vi "CANFD Frame to std frm.vi"(1 "Channel":i32, 3 "CANFD Frame":T2(array[cluster])) -> (0 "CAN Std Frm":T1[](array[typedef]) {"Direction" items=["Tx", "Rx"]; "CANType" items=["CAN", "CANFD", "CANFD加速"]})   [LabVIEW 2018, in "CAN FD.lvlib"]
uses:
  CAN FD.lvlib
  Typedef/CAN Data.ctl
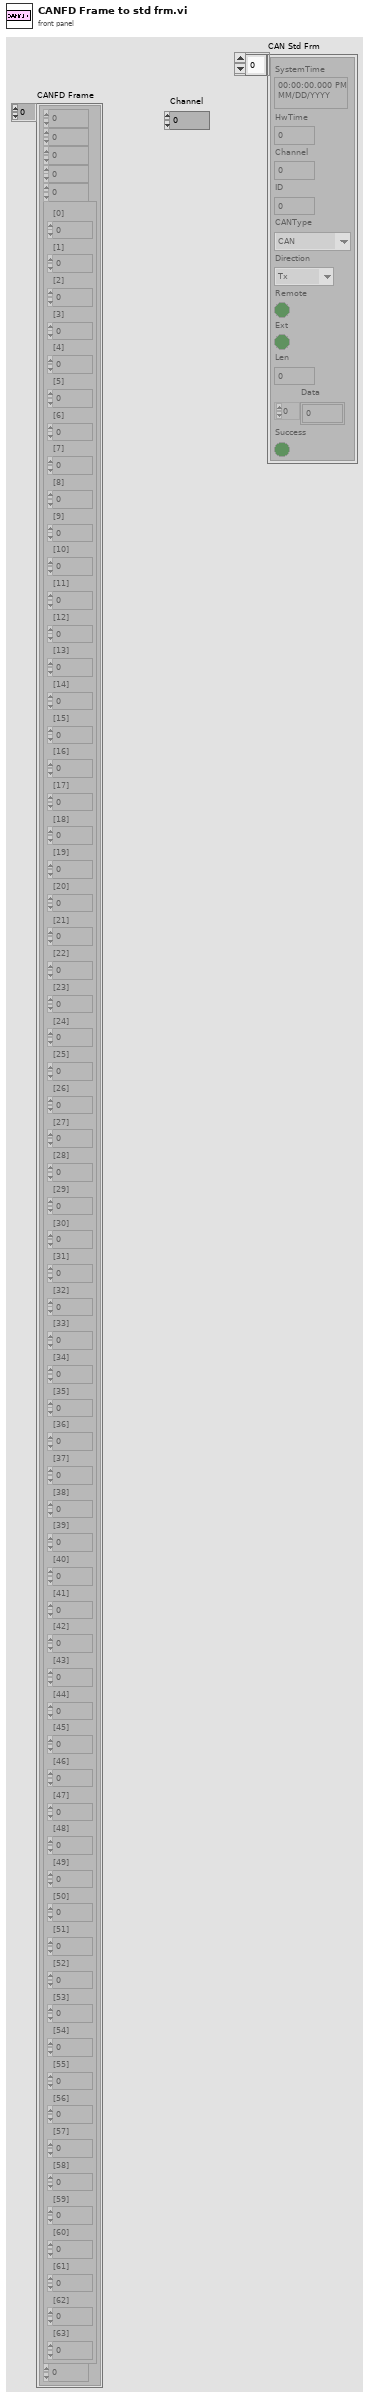
[diagram p1: front panel]
types:
  T1 = typedef "CAN FD.lvlib/CAN Data.ctl" = cluster{"SystemTime":timestamp, "HwTime":dbl, "Channel":u8, "ID":u32, "CANType":i16, "Direction":i16, "Remote":bool, "Ext":bool, "Len":u8, "Data":u8[], "Success":bool}
  T2 = cluster{u32, u8, u8, u8, u8, cluster{"[0]":u8, "[1]":u8, "[2]":u8, "[3]":u8, "[4]":u8, "[5]":u8, "[6]":u8, "[7]":u8, "[8]":u8, "[9]":u8, "[10]":u8, "[11]":u8, "[12]":u8, "[13]":u8, "[14]":u8, "[15]":u8, "[16]":u8, "[17]":u8, "[18]":u8, "[19]":u8, "[20]":u8, "[21]":u8, "[22]":u8, "[23]":u8, "[24]":u8, "[25]":u8, "[26]":u8, "[27]":u8, "[28]":u8, "[29]":u8, "[30]":u8, "[31]":u8, "[32]":u8, "[33]":u8, "[34]":u8, "[35]":u8, "[36]":u8, "[37]":u8, "[38]":u8, "[39]":u8, "[40]":u8, "[41]":u8, "[42]":u8, "[43]":u8, "[44]":u8, "[45]":u8, "[46]":u8, "[47]":u8, "[48]":u8, "[49]":u8, "[50]":u8, "[51]":u8, "[52]":u8, "[53]":u8, "[54]":u8, "[55]":u8, "[56]":u8, "[57]":u8, "[58]":u8, "[59]":u8, "[60]":u8, "[61]":u8, "[62]":u8, "[63]":u8}, u64}[]
  T3 = cluster{"[0]":u8, "[1]":u8, "[2]":u8, "[3]":u8, "[4]":u8, "[5]":u8, "[6]":u8, "[7]":u8, "[8]":u8, "[9]":u8, "[10]":u8, "[11]":u8, "[12]":u8, "[13]":u8, "[14]":u8, "[15]":u8, "[16]":u8, "[17]":u8, "[18]":u8, "[19]":u8, "[20]":u8, "[21]":u8, "[22]":u8, "[23]":u8, "[24]":u8, "[25]":u8, "[26]":u8, "[27]":u8, "[28]":u8, "[29]":u8, "[30]":u8, "[31]":u8, "[32]":u8, "[33]":u8, "[34]":u8, "[35]":u8, "[36]":u8, "[37]":u8, "[38]":u8, "[39]":u8, "[40]":u8, "[41]":u8, "[42]":u8, "[43]":u8, "[44]":u8, "[45]":u8, "[46]":u8, "[47]":u8, "[48]":u8, "[49]":u8, "[50]":u8, "[51]":u8, "[52]":u8, "[53]":u8, "[54]":u8, "[55]":u8, "[56]":u8, "[57]":u8, "[58]":u8, "[59]":u8, "[60]":u8, "[61]":u8, "[62]":u8, "[63]":u8}
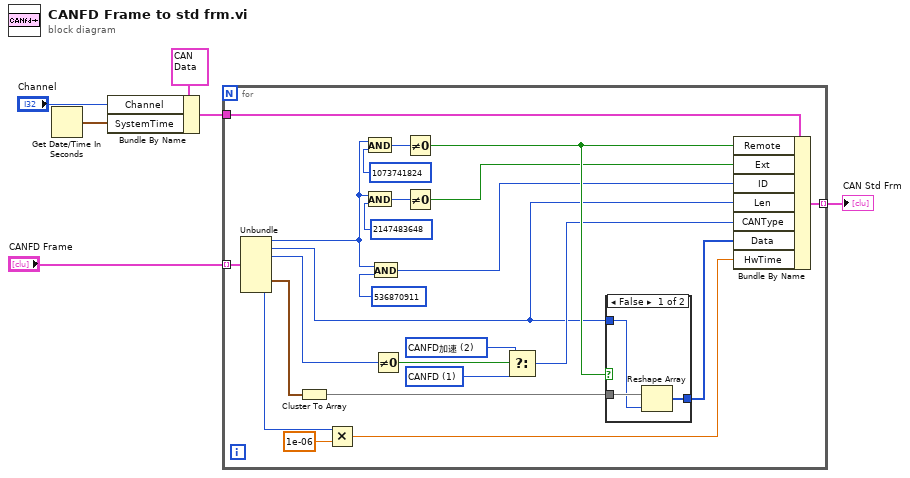
[diagram p0: block diagram]
diagram:
  n1 = Get Date/Time In Seconds() -> (seconds since 1Jan1904=w6:timestamp)
  n2 = Bundle By Name(cluster=T1 {"SystemTime"=timestamp(0 s since 1904-01-01), "HwTime"=0.0, "Channel"=0, "ID"=0, "CANType"=1, "Direction"=1, "Remote"=FALSE, "Ext"=FALSE, "Len"=0, "Data"=[], "Success"=FALSE} ("Data"), "Channel"="Channel", "SystemTime"=w6) -> (w3:T1)
  n3 = for {
    tunnel: "CANFD Frame" -> [w22] mode=indexing
    tunnel: w3 -> [w19]
    tunnel: [w8] -> w2 mode=indexing
    w14 = i16 1 items=["CAN", "CANFD", "CANFD加速"] ("CANType")
    w15 = i16 2 items=["CAN", "CANFD", "CANFD加速"] ("CANType")
    n4 = Unbundle(w22) -> (w25:u32, w7:u8, w21:u8, w24:T3, w10:u64)  [unwired: 2 out]
    n5 = Cluster To Array(cluster=w24) -> (array=w23:u8[])
    n6 = Multiply(x=w10, y=1e-06) -> (x*y=w9:dbl)
    n7 = And(x=w25, y=u32 1073741824) -> (x .and. y?=w26:u32)
    n8 = And(x=w25, y=u32 2147483648) -> (x .and. y?=w27:u32)
    n9 = And(x=w25, y=u32 536870911) -> (x .and. y?=w16:u32)
    n10 = Not Equal To 0?(x=w21) -> (x != 0?=w20:bool)
    n11 = Not Equal To 0?(x=w26) -> (x != 0?=w18:bool)
    n12 = Not Equal To 0?(x=w27) -> (x != 0?=w17:bool)
    n13 = Select(t=w15, s=w20, f=w14) -> (s? t:f=w13:i16)
    n14 = case shown="False" w18 {
      tunnel: [w32 _] -> w12
      tunnel: w23 -> [w33 _]
      tunnel: w7 -> [w31 _]
      frame False {
        n15 = Reshape Array(w33, w31) -> (w32:u8[])
      }
      frame True {
      }
    }
    n16 = Bundle By Name(cluster=w19, "Remote"=w18, "Ext"=w17, "ID"=w16, "Len"=w7, "CANType"=w13, "Data"=w12, "HwTime"=w9) -> (w8:T1)
  }
  "CAN Std Frm" <- w2
